vi "Save data.vi"() -> ()   [LabVIEW 2013]
panel:
  in  "파일 경로(대화 상자 사용)":path
  out "숫자형":i32
  out "All Data Graph 2":dbl[][](graph)
  in  "대기 시간(ms)":u32=1000
  in  "정지":bool
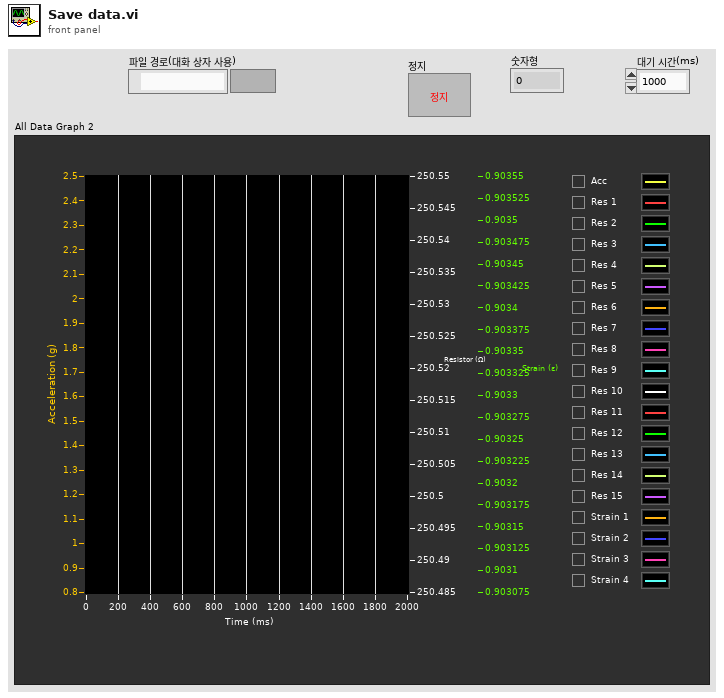
[diagram p1: front panel]
types:
  T1 = enum16{"open", "replace", "create", "open or create", "replace or create", "replace or create with confirmation"}
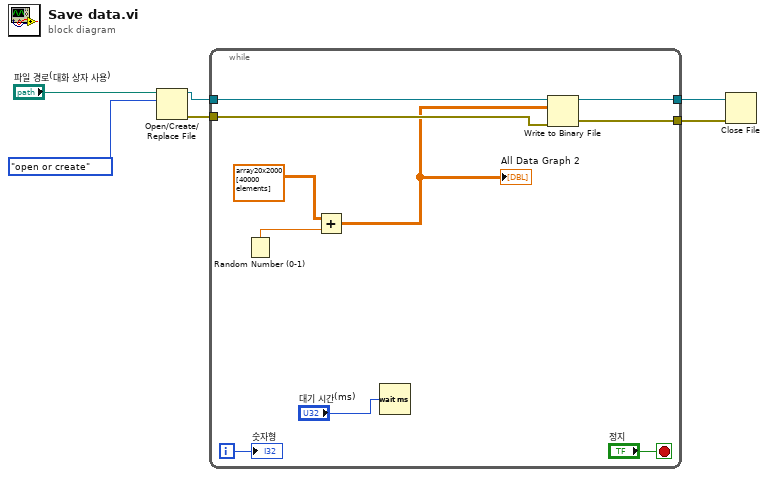
[diagram p0: block diagram]
diagram:
  n1 = Open/Create/Replace File(file path (use dialog)="파일 경로(대화 상자 사용)", operation (0:open)=T1."open or create" ("동작(0:open)")) -> (refnum out=w4:refnum<file>, error out=w5:errorcluster)  [unwired: 4 in, 1 out]
  n2 = while {
    tunnel: w5 -> [w11]
    tunnel: w4 -> [w10]
    tunnel: [w9] -> w3
    tunnel: [w8] -> w2
    i -> [w12]
    stop <- "정지" stop-if-true
    n3 = Random Number (0-1)() -> (number: 0 to 1=w16:dbl)
    n4 = Add(x=dbl[][] array20x2000[40000 elements] ("All Data Graph"), y=w16) -> (x+y=w7:dbl[][])
    "All Data Graph 2" <- w7
    n5 = Wait (ms)(milliseconds to wait="대기 시간(ms)") -> ()  [unwired: 1 out]
    n6 = Write to Binary File(file (use dialog)=w10, data=w7, error in=w11) -> (refnum out=w8:refnum<file>, error out=w9:errorcluster)  [unwired: 3 in, 1 out]
    "숫자형" <- w12
  }
  n7 = Close File(refnum=w2, error in=w3) -> ()  [unwired: 2 out]
